vi "Pause RS485.vi"(8 "error in (no error)":errorcluster, 10 "Internal?":bool, 11 "Huber Unistat 410 Settings":T1 {"Address" min=0 max=99 format="%02.0f"}) -> (0 "error out":errorcluster, 3 "Huber Unistat 410 Settings":T1 {"Address" min=0 max=99 format="%02.0f"})   [LabVIEW 2021, in "Huber Unistat 410 TCU.lvlib"]
uses:
  Huber Unistat 410 TCU.lvlib
  Huber Unistat 410 RS485 Settings.ctl
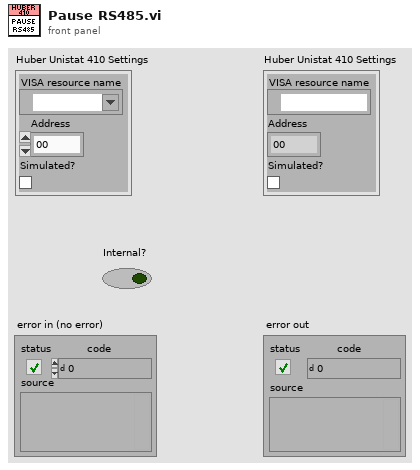
[diagram p1: front panel]
types:
  T1 = typedef "Huber Unistat 410 TCU.lvlib/Huber Unistat 410 RS485 Settings.ctl" = cluster{"VISA resource name":refnum<visa-resource-name>, "Address":i8, "Simulated?":bool}
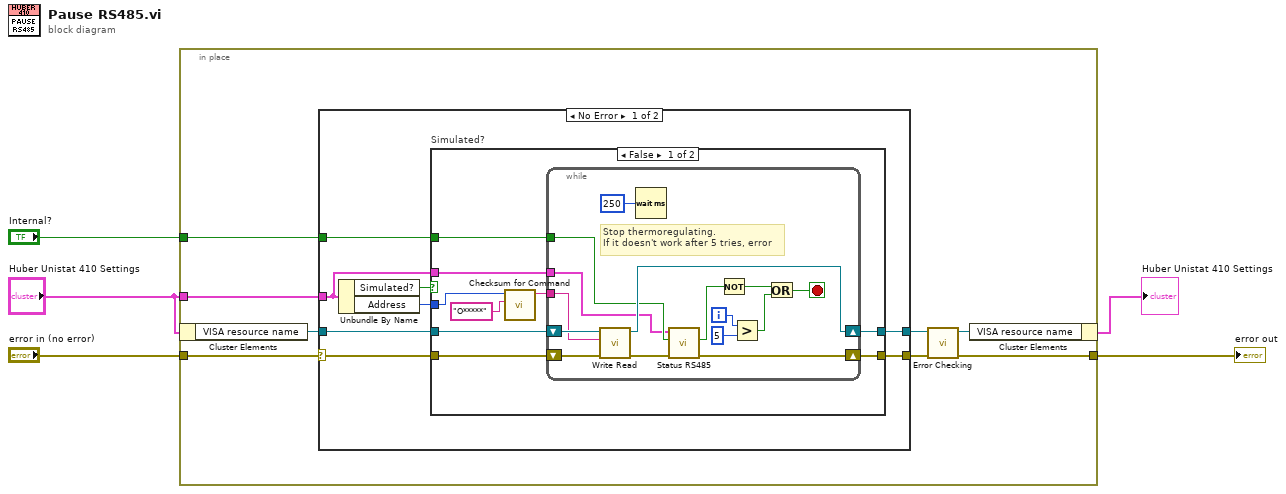
[diagram p0: block diagram]
diagram:
  n1 = in-place {
    in-place-border: "error in (no error)" -> [w13]
    in-place-border: [w10] -> w4
    in-place-border: "Huber Unistat 410 Settings" -> [w9]
    in-place-border: "Internal?" -> [w8]
    n2 = in-place-cluster #1("Huber Unistat 410 Settings") -> ("VISA resource name"=w7:refnum<visa-resource-name>)
    n3 = case shown="No Error" w13 {
      selector: w13 -> [w21 w49]
      tunnel: w9 -> [w17 _]
      tunnel: [w20 w49] -> w11
      tunnel: [w19 w48] -> w12
      tunnel: w8 -> [w16 _]
      tunnel: w7 -> [w15 w48]
      frame No Error {
        n4 = Unbundle By Name(w17) -> ("Simulated?"=w18:bool, "Address"=w14:i8)
        n5 = case "Simulated?" shown="False" w18 {
          tunnel: w21 -> [w28 w47]
          tunnel: [w26 w47] -> w20
          tunnel: [w30 w46] -> w19
          tunnel: w15 -> [w29 w46]
          tunnel: w17 -> [w27 _]
          tunnel: w16 -> [w25 _]
          tunnel: w14 -> [w24 _]
          frame False {
            n6 = call "Checksum for Command.vi"("Message"="O*****" ("string"), "Address"=w24) -> ("Formated Message"=w22:string)  [unwired: 9 in]
            n7 = while {
              tunnel: w27 -> [w32]
              shift-right: [w38] -> w30
              shift-left: w29 -> [w40]
              shift-right: [w35] -> w26
              shift-left: w28 -> [w39]
              tunnel: w25 -> [w33]
              tunnel: w22 -> [w31]
              i -> [w44]
              stop <- w45 stop-if-true
              # "Stop thermoregulating. \nIf it doesn't work after 5 tries, error"
              n8 = call "Write Read.vi"("error in (no error)"=w39, "write string"=w31, "VISA Refnum in"=w40) -> ("error out"=w34:errorcluster, "VISA Refnum out"=w38:refnum<visa-resource-name>)  [unwired: 6 in, 1 out]
              n9 = Wait (ms)(milliseconds to wait=u32 250) -> ()  [unwired: 1 out]
              n10 = call "Status RS485.vi"("error in (no error)"=w34, "Internal?"=w33, "Huber Unistat 410 Settings"=w32) -> ("error out"=w35:errorcluster, "Running"=w36:bool)  [unwired: 4 in, 3 out]
              n11 = Not(x=w36) -> (.not. x?=w37:bool)
              n12 = Greater?(x=w44, y=5) -> (0:w42:bool)
              n13 = Or(x=w37, y=w42) -> (x .or. y?=w45:bool)
            }
          }
          frame True {
          }
        }
      }
      frame Error {
      }
    }
    n14 = call "Error Checking.vi"("error in (no error)"=w11, "VISA resource name"=w12) -> ("error out"=w10:errorcluster, "VISA resource name"=w6:refnum<visa-resource-name>)  [unwired: 7 in, 1 out]
    n15 = in-place-cluster #1("VISA resource name"=w6) -> (→"Huber Unistat 410 Settings":T1)
  }
  "error out" <- w4
